vi "HFRR ADV v04.vi"() -> ()   [LabVIEW 2025] (continued)
                w1869 = FALSE ("autostrtflg")
                n931 = local write "autostrtflg"(w1869) -> ()
                n932 = local write "autostart"(w1869) -> ()
                n933 = local write "RUN"(TRUE ("RUN")) -> ()
                n934 = local write "String 14"(" Running....." ("String 14")) -> ()
              }
            }
          }
          frame Enabled {
          }
        }
        n935 = Insert Into Array(array=string[] ["Air Temperature has reached set value,", "Humidity has reached set value,", "Sample Temperaturehas reached set value,", ""], index=0, new element="") -> (w1820:string[])
        n936 = for {
          tunnel: w1821 -> [w1919] mode=indexing
          tunnel: w1820 -> [w1918]
          shift-right: [w1915] -> w1819
          shift-left: "" -> [w1917]
          n937 = Index Array(array=w1918, index=w1919) -> (element=w1916:string)
          n938 = Concatenate Strings(w1916, w1917) -> (w1915:string)
        }
        n939 = local write "autostart 2"(w1819) -> ()
      }
      frame 1 {
        # "Elapsed time\ncof\nstroke\nAir temp\nTemp\nHumidity"
        n940 = case shown="True" "OPEN 4" {
          frame False {
          }
          frame True {
            (unwired) 0  # existing file
            w2428 = "Choose a datalog file to open"  # prompt
            n941 = local write "OPEN 4"(FALSE ("OPEN 1")) -> ()
            n942 = String To Path(string="C:\\LAB-IQ-NXT\\Data\\") -> (path=w2413:path)
            n943 = File Dialog(6:"*.dgf" ("pattern"), 7:w2428, 11:w2413) -> (0:w2411:errorcluster, 3:w2419:path)  [unwired: 4 in, 2 out]
            n944 = Unbundle(w2411) -> ()  [unwired: 3 out]
            n945 = Path To String(path=w2419) -> (string=w2414:string)
            "string1 4" <- w2414
            n946 = Match Pattern(string=w2414, regular expression=".dgf" ("substring (\"\")")) -> (before substring=w2424:string)  [unwired: 1 in, 3 out]
            n947 = Concatenate Strings(w2424, ".duf" ("Substring")) -> (w2421:string)
            n948 = String To Path(string=w2421) -> (path=w2425:path)
            n949 = call <vilib>:"Read Characters From File.vi"("file path (dialog if empty)"=w2425, "start of read offset (chars.:0)"=60 ("start of read offset (chars.: 0)")) -> ("character string"=→"String Control 8":string)  [unwired: 4 in, 3 out]
            n950 = Strip Path(path=w2419) -> (name=w2417:string)  [unwired: 1 out]
            n951 = Match Pattern(string=w2417, regular expression=".dgf") -> (before substring=→"String Control 7":string)  [unwired: 1 in, 3 out]
          }
        }
        n952 = case shown="True" "OPEN 3" {
          frame False {
          }
          frame True {
            (unwired) 0  # existing file
            w2410 = "Choose a datalog file to open"  # prompt
            n953 = local write "OPEN 3"(FALSE ("OPEN 1")) -> ()
            n954 = String To Path(string="C:\\LAB-IQ-NXT\\Data\\") -> (path=w2395:path)
            n955 = File Dialog(6:"*.dgf" ("pattern"), 7:w2410, 11:w2395) -> (0:w2393:errorcluster, 3:w2401:path)  [unwired: 4 in, 2 out]
            n956 = Unbundle(w2393) -> ()  [unwired: 3 out]
            n957 = Path To String(path=w2401) -> (string=w2396:string)
            "string1 3" <- w2396
            n958 = Match Pattern(string=w2396, regular expression=".dgf" ("substring (\"\")")) -> (before substring=w2406:string)  [unwired: 1 in, 3 out]
            n959 = Concatenate Strings(w2406, ".duf" ("Substring")) -> (w2403:string)
            n960 = String To Path(string=w2403) -> (path=w2407:path)
            n961 = call <vilib>:"Read Characters From File.vi"("file path (dialog if empty)"=w2407, "start of read offset (chars.:0)"=60 ("start of read offset (chars.: 0)")) -> ("character string"=→"String Control 6":string)  [unwired: 4 in, 3 out]
            n962 = Strip Path(path=w2401) -> (name=w2399:string)  [unwired: 1 out]
            n963 = Match Pattern(string=w2399, regular expression=".dgf") -> (before substring=→"String Control 5":string)  [unwired: 1 in, 3 out]
          }
        }
        n964 = case shown="True" "OPEN 2" {
          frame False {
          }
          frame True {
            (unwired) 0  # existing file
            w2392 = "Choose a datalog file to open"  # prompt
            n965 = local write "OPEN 2"(FALSE ("OPEN 1")) -> ()
            n966 = String To Path(string="C:\\LAB-IQ-NXT\\Data\\") -> (path=w2377:path)
            n967 = File Dialog(6:"*.dgf" ("pattern"), 7:w2392, 11:w2377) -> (0:w2375:errorcluster, 3:w2383:path)  [unwired: 4 in, 2 out]
            n968 = Unbundle(w2375) -> ()  [unwired: 3 out]
            n969 = Path To String(path=w2383) -> (string=w2378:string)
            "string1 2" <- w2378
            n970 = Match Pattern(string=w2378, regular expression=".dgf" ("substring (\"\")")) -> (before substring=w2389:string)  [unwired: 1 in, 3 out]
            n971 = Concatenate Strings(w2389, ".duf" ("Substring")) -> (w2386:string)
            n972 = String To Path(string=w2386) -> (path=w2384:path)
            n973 = call <vilib>:"Read Characters From File.vi"("file path (dialog if empty)"=w2384, "start of read offset (chars.:0)"=60 ("start of read offset (chars.: 0)")) -> ("character string"=→"String Control 4":string)  [unwired: 4 in, 3 out]
            n974 = Strip Path(path=w2383) -> (name=w2381:string)  [unwired: 1 out]
            n975 = Match Pattern(string=w2381, regular expression=".dgf") -> (before substring=→"String Control 3":string)  [unwired: 1 in, 3 out]
          }
        }
        n976 = case shown="True" "OPEN 1" {
          frame False {
          }
          frame True {
            (unwired) 0  # existing file
            w2374 = "Choose a datalog file to open"  # prompt
            n977 = local write "OPEN 1"(FALSE ("OPEN 1")) -> ()
            n978 = String To Path(string="C:\\LAB-IQ-NXT\\Data\\") -> (path=w2359:path)
            n979 = File Dialog(6:"*.dgf" ("pattern"), 7:w2374, 11:w2359) -> (0:w2357:errorcluster, 3:w2365:path)  [unwired: 4 in, 2 out]
            n980 = Unbundle(w2357) -> ()  [unwired: 3 out]
            n981 = Path To String(path=w2365) -> (string=w2360:string)
            "string1" <- w2360
            n982 = Match Pattern(string=w2360, regular expression=".dgf" ("substring (\"\")")) -> (before substring=w2370:string)  [unwired: 1 in, 3 out]
            n983 = Concatenate Strings(w2370, ".duf" ("Substring")) -> (w2366:string)
            n984 = String To Path(string=w2366) -> (path=w2371:path)
            n985 = call <vilib>:"Read Characters From File.vi"("file path (dialog if empty)"=w2371, "start of read offset (chars.:0)"=60 ("start of read offset (chars.: 0)")) -> ("character string"=→"String Control 2":string)  [unwired: 4 in, 3 out]
            n986 = Strip Path(path=w2365) -> (name=w2364:string)  [unwired: 1 out]
            n987 = Match Pattern(string=w2364, regular expression=".dgf") -> (before substring=→"String Control":string)  [unwired: 1 in, 3 out]
          }
        }
        n988 = case shown="True" "RSTV1 4" {
          frame False {
          }
          frame True {
            n989 = property on="Stroke" class="XYGraph (strict)"("Y Scale.Display Format:Precision"=u8 2 ("Y Scale.Format & Precision:Precision")) -> ()  [unwired: 2 in, 2 out]
            n990 = property on="Stroke" class="XYGraph (strict)"("X Scale.Range:Minimum"=0.0 ("Y Scale.Range:Maximum"), "X Scale.Range:Maximum"=75.0 ("X Scale.Range:Minimum"), "Y Scale.Range:Minimum"=0.98, "Y Scale.Range:Maximum"=1.02) -> ()  [unwired: 2 in, 2 out]
          }
        }
        n991 = case shown="True" "rstv2" {
          frame False {
          }
          frame True {
            n992 = property on="Coefficient Of Friction" class="XYGraph (strict)"("X Scale.Range:Minimum"=0.0 ("Y Scale.Range:Maximum"), "X Scale.Range:Maximum"=75.0, "Y Scale.Range:Minimum"=0.0, "Y Scale.Range:Maximum"=1.0 ("X Scale.Range:Minimum")) -> ()  [unwired: 2 in, 2 out]
            n993 = property on="Coefficient Of Friction" class="XYGraph (strict)"("Y Scale.Display Format:Precision"=u8 3 ("Y Scale.Format & Precision:Precision")) -> ()  [unwired: 2 in, 2 out]
          }
        }
        n994 = case shown="True" "RSTV1 3" {
          frame False {
          }
          frame True {
            n995 = property on="Air Temperature" class="XYGraph (strict)"("X Scale.Range:Minimum"=0.0 ("Y Scale.Range:Minimum"), "X Scale.Range:Maximum"=75.0 ("Y Scale.Range:Maximum"), "Y Scale.Range:Minimum"=20.0 ("X Scale.Range:Minimum"), "Y Scale.Range:Maximum"=26.0 ("X Scale.Range:Maximum")) -> ()  [unwired: 2 in, 2 out]
            n996 = property on="Air Temperature" class="XYGraph (strict)"("Y Scale.Display Format:Precision"=u8 2 ("Y Scale.Format & Precision:Precision")) -> ()  [unwired: 2 in, 2 out]
          }
        }
        n997 = case shown="True" "RST CP" {
          frame False {
          }
          frame True {
            n998 = property on="Sample Temperature" class="XYGraph (strict)"("X Scale.Range:Minimum"=0.0, "X Scale.Range:Maximum"=75.0, "Y Scale.Range:Minimum"=58.0, "Y Scale.Range:Maximum"=62.0) -> ()  [unwired: 2 in, 2 out]
            n999 = property on="Sample Temperature" class="XYGraph (strict)"("Y Scale.Display Format:Precision"=u8 2 ("Y Scale.Format & Precision:Precision")) -> ()  [unwired: 2 in, 2 out]
          }
        }
        n1000 = case shown="True" "RST CP 2" {
          frame False {
          }
          frame True {
            n1001 = property on="XY Graph 13" class="XYGraph (strict)"("X Scale.Range:Minimum"=0.0, "X Scale.Range:Maximum"=75.0, "Y Scale.Range:Minimum"=0.0, "Y Scale.Range:Maximum"=100.0) -> ()  [unwired: 2 in, 2 out]
            n1002 = property on="XY Graph 13" class="XYGraph (strict)"("Y Scale.Display Format:Precision"=u8 0 ("Y Scale.Format & Precision:Precision")) -> ()  [unwired: 2 in, 2 out]
          }
        }
        n1003 = case shown="True" "RSTV1 2" {
          frame False {
          }
          frame True {
            n1004 = property on="Humidity" class="XYGraph (strict)"("X Scale.Range:Minimum"=0.0, "X Scale.Range:Maximum"=75.0, "Y Scale.Range:Minimum"=48.0, "Y Scale.Range:Maximum"=58.0) -> ()  [unwired: 2 in, 2 out]
            n1005 = property on="Humidity" class="XYGraph (strict)"("Y Scale.Display Format:Precision"=u8 0 ("Y Scale.Format & Precision:Precision")) -> ()  [unwired: 2 in, 2 out]
          }
        }
        n1006 = case shown="True" "RST CP 3" {
          frame False {
          }
          frame True {
            n1007 = property on="Air Temp vs Rh" class="XYGraph (strict)"("X Scale.Range:Minimum"=18.0, "X Scale.Range:Maximum"=28.0 ("X Scale.Range:Minimum"), "Y Scale.Range:Minimum"=30.0 ("X Scale.Range:Minimum"), "Y Scale.Range:Maximum"=70.0 ("X Scale.Range:Minimum")) -> ()  [unwired: 2 in, 2 out]
          }
        }
      }
      frame 2 {
        # "Elapsed time\ncof\nstroke\nmean pos\nTemp\nHumidity"
        n1008 = case shown="True" "Export" {
          frame False {
          }
          frame True {
            w2558 = "                                      " ("string")
            w2560 = "\r"
            (unwired) i16 6 ("width (-)")
            w2637 = "\r"
            w2569 = "\r"
            n1009 = local read "Sample ID"() -> (w2644:string)
            n1010 = local read "Temperature after test 2"() -> (w2631:dbl)
            n1011 = local read "Test Date"() -> (w2643:string)
            n1012 = local read "String 45"() -> (w2557:string)
            n1013 = local read "String 32"() -> (w2641:string)
            n1014 = local read "String 31"() -> (w2642:string)
            n1015 = local read "String 38"() -> (w2579:string)
            n1016 = local read "Humidity after test 2"() -> (w2627:dbl)
            n1017 = local read "s.NO"() -> (w2559:string)
            n1018 = local read "String 36"() -> (w2582:string)
            n1019 = local read "Temperature before test 2"() -> (w2626:dbl)
            n1020 = local read "String 37"() -> (w2585:string)
            n1021 = local read "AVP 2"() -> (w2624:dbl)
            n1022 = local read "HCF 2"() -> (w2635:dbl)
            n1023 = local read "MWSD 2"() -> (w2623:dbl)
            n1024 = local read "String 35"() -> (w2589:string)
            n1025 = local write "Export"(FALSE ("Export")) -> ()
            n1026 = local read "Humidity before test 2"() -> (w2612:dbl)
            n1027 = Concatenate Strings("7," ("string"), w2579) -> (w2580:string)
            n1028 = Concatenate Strings("6," ("string"), w2582) -> (w2583:string)
            n1029 = local read "S 39"() -> (w2590:string)
            n1030 = Concatenate Strings("5," ("string"), w2585) -> (w2586:string)
            n1031 = local read "String 34"() -> (w2594:string)
            n1032 = Concatenate Strings("4," ("string"), w2589) -> (w2588:string)
            n1033 = Concatenate Strings("3," ("string"), w2590) -> (w2592:string)
            n1034 = local read "S 38"() -> (w2597:string)
            n1035 = Number To Fractional String(number=w2635, width (-)=i16 6, precision (6)=i16 2) -> (F-format string=w2636:string)  [unwired: 1 in]
            n1036 = Number To Fractional String(number=w2623, width (-)=i16 6, precision (6)=i16 2) -> (F-format string=w2621:string)  [unwired: 1 in]
            n1037 = Number To Fractional String(number=w2624, width (-)=i16 6, precision (6)=i16 2) -> (F-format string=w2622:string)  [unwired: 1 in]
            n1038 = Number To Fractional String(number=w2631, width (-)=i16 6, precision (6)=i16 2) -> (F-format string=w2630:string)  [unwired: 1 in]
            n1039 = Number To Fractional String(number=w2627, width (-)=i16 6, precision (6)=i16 2) -> (F-format string=w2625:string)  [unwired: 1 in]
            n1040 = Number To Fractional String(number=w2626, width (-)=i16 6, precision (6)=i16 2) -> (F-format string=w2632:string)  [unwired: 1 in]
            n1041 = Number To Fractional String(number=w2612, width (-)=i16 6, precision (6)=i16 2) -> (F-format string=w2611:string)  [unwired: 1 in]
            n1042 = local read "String 39"() -> (w2576:string)
            n1043 = Concatenate Strings("2," ("string"), w2594) -> (w2593:string)
            n1044 = local read "WS1.4 2"() -> (w2639:dbl)
            n1045 = Concatenate Strings(w2569, "," ("string"), w2557, w2559, w2558, w2641, w2644, w2558, w2642, w2643, w2569) -> (w2567:string)
            n1046 = Concatenate Strings("1," ("string"), w2597) -> (w2596:string)
            n1047 = Concatenate Strings("8," ("string"), w2576) -> (w2577:string)
            n1048 = Number To Fractional String(number=w2639, precision (6)=i16 2) -> (F-format string=w2640:string)  [unwired: 2 in]
            n1049 = Concatenate Strings(w2637, w2596, w2611, w2637, w2593, w2632, w2637, w2592, w2625, w2637, w2588, w2630, w2637, w2586, w2621, w2637, w2583, w2622, w2637, w2580, w2636, w2637, w2577, w2640) -> (w2599:string)
            n1050 = Concatenate Strings("S.No," ("string"), "                                       Parameters" ("string")) -> (w2570:string)
            n1051 = local read "TITTLE"() -> (w2565:string)
            n1052 = local read "String 33"() -> (w2574:string)
            n1053 = local read "Tested by"() -> (w2573:string)
            n1054 = Concatenate Strings("=" ("string"), w2565) -> (w2564:string)
            n1055 = local read "String 29"() -> (w2606:string)
            n1056 = Concatenate Strings("," ("string"), "                                                                             " ("string")) -> (w2562:string)
            n1057 = Concatenate Strings(w2564, w2560, w2567, w2560, w2570, w2599, w2560, w2562, w2574, w2573) -> (→"export":string)
            n1058 = Match Pattern(string=w2606, regular expression=".dwm") -> (before substring=w2602:string)  [unwired: 1 in, 3 out]
            "before substring" <- w2602
            n1059 = case shown="\"xlx\"" "Select File Type" {
              tunnel: w2602 -> [w2647 w2649 w2651]
              tunnel: [w2645 w2650 w2652] -> w2601
              frame "xlx" {
                n1060 = Concatenate Strings(w2647, ".xls" ("string")) -> (w2645:string)
              }
              frame "csv" {
                n1061 = Concatenate Strings(w2649, ".csv" ("string")) -> (w2650:string)
              }
              frame "txt" {
                n1062 = Concatenate Strings(w2651, ".txt" ("string")) -> (w2652:string)
              }
            }
            n1063 = String To Path(string=w2601) -> (path=w2608:path)
            n1064 = local read "export"() -> (w2603:string)
            n1065 = call <vilib>:"Write Characters To File.vi"("append to file? (new file:F)"=FALSE, "character string"=w2603, "file path (dialog if empty)"=w2608) -> ()  [unwired: 2 in, 1 out]
          }
        }
        n1066 = case shown="True" "OK Button 16" {
          frame False {
          }
          frame True {
            n1067 = stacked-sequence {
              frame #0 {
                n1068 = local read "Numeric 16"() -> (w2767:i32)
                n1069 = local write "Numeric 10"(w2767) -> ()
              }
              frame #1 {
                n1070 = local read "String 29"() -> (w2771:string)
                n1071 = String To Path(string=w2771) -> (path=w2770:path)
                n1072 = local read "S.NO"() -> (→"s.NO":string)
                n1073 = Open/Create/Replace File "Open File"(file path (use dialog)=w2770) -> (refnum out=w2772:refnum<file>)  [unwired: 5 in, 2 out]
                n1074 = for {
                  N: 16 -> [_]
                  tunnel: w2772 -> [w2779]
                  i -> [w2775]
                  (unwired) TRUE ("line mode (F)")
                  n1075 = Read from Text File "Read File"(file (use dialog)=w2779) -> (text=w2773:string)  [unwired: 3 in, 3 out]
                  n1076 = Match Pattern(string=w2773, regular expression="(") -> (after substring=w2778:string)  [unwired: 1 in, 3 out]
                  n1077 = Match Pattern(string=w2778, regular expression=")") -> (before substring=w2774:string)  [unwired: 1 in, 3 out]
                  n1078 = case shown="1" w2775 {
                    tunnel: w2774 -> [w2780 w2781 _ _ w2782 w2783 w2784 w2786 w2788 w2790 w2792 w2794 w2796 w2798 _]
                    tunnel: w2773 -> [_ _ _ _ _ _ _ _ _ _ _ _ _ _ _]
                    frame 0 {
                      "TITTLE" <- w2780
                    }
                    frame 1 {
                      "Sample ID" <- w2781
                    }
                    frame 2 {
                    }
                    frame 3 {
                    }
                    frame 4 {
                      "Test Date" <- w2782
                    }
                    frame 5 {
                      "Tested by" <- w2783
                    }
                    frame 6 {
                      n1079 = Fract/Exp String To Number(string=w2784) -> (number=→"Humidity before test 2":dbl)  [unwired: 3 in, 1 out]
                    }
                    frame 7 {
                      n1080 = Fract/Exp String To Number(string=w2786) -> (number=→"Temperature before test 2":dbl)  [unwired: 3 in, 1 out]
                    }
                    frame 8 {
                      n1081 = Fract/Exp String To Number(string=w2788) -> (number=→"Humidity after test 2":dbl)  [unwired: 3 in, 1 out]
                    }
                    frame 9 {
                      n1082 = Fract/Exp String To Number(string=w2790) -> (number=→"Temperature after test 2":dbl)  [unwired: 3 in, 1 out]
                    }
                    frame 10 {
                      n1083 = Fract/Exp String To Number(string=w2792) -> (number=→"MWSD 2":dbl)  [unwired: 3 in, 1 out]
                    }
                    frame 11 {
                      n1084 = Fract/Exp String To Number(string=w2794) -> (number=→"AVP 2":dbl)  [unwired: 3 in, 1 out]
                    }
                    frame 12 {
                      n1085 = Fract/Exp String To Number(string=w2796) -> (number=→"HCF 2":dbl)  [unwired: 3 in, 1 out]
                    }
                    frame 13 {
                      n1086 = Fract/Exp String To Number(string=w2798) -> (number=→"WS1.4 2":dbl)  [unwired: 3 in, 1 out]
                    }
                    frame 14, Default {
                    }
                  }
                }
              }
              frame #2 {
              }
            }
            n1087 = local write "OK Button 16"(FALSE ("OK Button 13")) -> ()
          }
        }
        n1088 = call <vilib>:"Query Available Printers.vi"() -> ("system configured printers"=w2443:string[])  [unwired: 9 in, 2 out]
        "System Configured Printers 2" <- w2443
        n1089 = Index Array(array=w2443, index="Select Printer 3") -> (element=w2445:string)
        "Selected Printer" <- w2445
        n1090 = local read "OK Button 16"() -> (w2439:bool)
        n1091 = case shown="True" "Print" {
          tunnel: w2445 -> [_ w2736]
          frame False {
          }
          frame True {
            (unwired) i16 6 ("width (-)")
            (unwired) "TESTED BY : "
            (unwired) "TESTED DATE :"
            (unwired) "SAMPLE ID : "
            (unwired) "SAMPLE DESIGN : "
            w2694 = "\r"
            w2711 = "\r"
            # "add image"
            n1092 = local read "String 45"() -> (w2654:string)
            n1093 = local read "Sample ID"() -> (w2684:string)
            n1094 = local read "Tested by"() -> (w2687:string)
            n1095 = local read "Test Date"() -> (w2685:string)
            n1096 = local read "String 32"() -> (w2689:string)
            n1097 = local read "String 31"() -> (w2688:string)
            n1098 = local read "String 33"() -> (w2690:string)
            n1099 = local read "s.NO"() -> (w2655:string)
            n1100 = call <vilib>:"New Report.vi"("report type"=enum16{"Standard Report", "HTML"}."Standard Report") -> ("report out"=w2734:refnum<class "NI_report.lvclass">, "error out"=w2733:errorcluster)  [unwired: 13 in]
            n1101 = local read "TITTLE"() -> (w2686:string)
            n1102 = call-dynamic "Set Report Header Text.vi"("report in"=w2734, "center header text"=w2686, "error in (no error)"=w2733) -> ("report out"=w2705:refnum<class "NI_report.lvclass">, "error out"=w2706:errorcluster)  [unwired: 11 in]
            n1103 = Concatenate Strings(w2711, w2654, w2655, w2711, w2689, w2684, w2711, w2688, w2685, w2711, w2690, w2687, w2711) -> (w2704:string)
            "test by" <- w2704
            n1104 = local read "Temperature after test 2"() -> (w2700:dbl)
            n1105 = local read "String 38"() -> (w2660:string)
            n1106 = local read "Humidity after test 2"() -> (w2709:dbl)
            n1107 = local read "String 36"() -> (w2664:string)
            n1108 = local read "Temperature before test 2"() -> (w2710:dbl)
            n1109 = local read "String 37"() -> (w2667:string)
            n1110 = local read "AVP 2"() -> (w2713:dbl)
            n1111 = local read "HCF 2"() -> (w2696:dbl)
            n1112 = local read "MWSD 2"() -> (w2714:dbl)
            n1113 = local read "String 35"() -> (w2669:string)
            n1114 = call-poly <vilib>:"Append Report Text.vi"("report in"=w2705, "text"=w2704, "error in (no error)"=w2706) -> ("report out"=w2708:refnum<class "NI_report.lvclass">, "error out"=w2707:errorcluster)  [unwired: 9 in, 2 out]
            n1115 = local read "Humidity before test 2"() -> (w2725:dbl)
            n1116 = Concatenate Strings("7)" ("string"), w2660) -> (w2661:string)
            n1117 = local read "S 39"() -> (w2672:string)
            n1118 = local read "String 34"() -> (w2674:string)
            n1119 = Concatenate Strings("6)" ("string"), w2664) -> (w2663:string)
            n1120 = Concatenate Strings("5)" ("string"), w2667) -> (w2666:string)
            n1121 = Concatenate Strings("4)" ("string"), w2669) -> (w2670:string)
            n1122 = Concatenate Strings("3)" ("string"), w2672) -> (w2673:string)
            n1123 = local read "S 38"() -> (w2679:string)
            n1124 = Concatenate Strings("2)" ("string"), w2674) -> (w2675:string)
            n1125 = Number To Fractional String(number=w2696, width (-)=i16 6, precision (6)=i16 2) -> (F-format string=w2695:string)  [unwired: 1 in]
            n1126 = Number To Fractional String(number=w2714, width (-)=i16 6, precision (6)=i16 2) -> (F-format string=w2716:string)  [unwired: 1 in]
            n1127 = Number To Fractional String(number=w2713, width (-)=i16 6, precision (6)=i16 2) -> (F-format string=w2715:string)  [unwired: 1 in]
            n1128 = Number To Fractional String(number=w2700, width (-)=i16 6, precision (6)=i16 2) -> (F-format string=w2701:string)  [unwired: 1 in]
            n1129 = Number To Fractional String(number=w2709, width (-)=i16 6, precision (6)=i16 2) -> (F-format string=w2712:string)  [unwired: 1 in]
            n1130 = Number To Fractional String(number=w2710, width (-)=i16 6, precision (6)=i16 2) -> (F-format string=w2699:string)  [unwired: 1 in]
            n1131 = Number To Fractional String(number=w2725, width (-)=i16 6, precision (6)=i16 2) -> (F-format string=w2730:string)  [unwired: 1 in]
            n1132 = call-poly <vilib>:"Append Report Text.vi"("report in"=w2708, "error in (no error)"=w2707) -> ("report out"=w2729:refnum<class "NI_report.lvclass">, "error out"=w2727:errorcluster)  [unwired: 10 in, 2 out]
            n1133 = local read "String 39"() -> (w2657:string)
            n1134 = local read "WS1.4 2"() -> (w2692:dbl)
            n1135 = Concatenate Strings("1)" ("string"), w2679) -> (w2678:string)
            n1136 = Concatenate Strings("8)" ("string"), w2657) -> (w2658:string)
            n1137 = Number To Fractional String(number=w2692, precision (6)=i16 2) -> (F-format string=w2691:string)  [unwired: 2 in]
            n1138 = Concatenate Strings(w2694, w2678, w2730, w2694, w2675, w2699, w2694, w2673, w2712, w2694, w2670, w2701, w2694, w2666, w2716, w2694, w2663, w2715, w2694, w2661, w2695, w2694, w2658, w2691) -> (w2682:string)
            "export 2" <- w2682
            n1139 = call-poly <vilib>:"Append Report Text.vi"("report in"=w2729, "text"=w2682, "error in (no error)"=w2727) -> ("report out"=w2728:refnum<class "NI_report.lvclass">, "error out"=w2726:errorcluster)  [unwired: 9 in, 2 out]
            n1140 = call-dynamic "Print Report.vi"("report in"=w2728, "printer name (default)"=w2736, "error in (no error)"=w2726) -> ("report out"=w2738:refnum<class "NI_report.lvclass">, "error out"=w2739:errorcluster)  [unwired: 11 in]
            n1141 = local read "test by"() -> (w2681:string)
            n1142 = local read "TITTLE"() -> (w2683:string)
            n1143 = local write "Print"(FALSE ("Print FF")) -> ()
            n1144 = call-dynamic "Dispose Report.vi"("report in"=w2738, "error in (no error)"=w2739) -> ()  [unwired: 13 in, 1 out]
            n1145 = Concatenate Strings(w2683, w2682, w2681) -> (→"output":string)
          }
        }
        n1146 = case shown="True" w2439 {
          frame False {
          }
          frame True {
            n1147 = flat-sequence {
              frame #0 {
              }
              frame #1 {
                n1148 = Wait (ms)(milliseconds to wait=u32 100) -> ()  [unwired: 1 out]
              }
              frame #2 {
                n1149 = local write "OK Button 16"(FALSE ("Print 3")) -> ()
              }
            }
          }
        }
        n1150 = case shown="True" "OK Button 17" {
          frame False {
          }
          frame True {
            (unwired) 0  # existing file
            w2753 = "Choose a datalog file to open"  # prompt
            n1151 = local read "String"() -> (w2748:string)
            n1152 = local write "OK Button 17"(FALSE ("OK Button 17")) -> ()
            n1153 = String To Path(string=w2748) -> (path=w2749:path)
            n1154 = File Dialog(6:"*.duf" ("pattern"), 7:w2753, 11:w2749) -> (0:w2740:errorcluster, 3:w2759:path)  [unwired: 4 in, 2 out]
            n1155 = Unbundle(w2740) -> ()  [unwired: 3 out]
            n1156 = Open/Create/Replace File "Open File"(file path (use dialog)=w2759) -> (refnum out=w2751:refnum<file>)  [unwired: 5 in, 2 out]
            n1157 = Path To String(path=w2759) -> (string=w2742:string)
            n1158 = while {
              tunnel: w2751 -> [w2763]
              i -> [w2760]
              stop <- w2761 continue-if-true
              (unwired) TRUE ("line mode (F)")
              n1159 = local write "Numeric 16"(w2760) -> ()
              n1160 = Read from Text File "Read File"(file (use dialog)=w2763) -> (text=w2762:string)  [unwired: 3 in, 3 out]
              n1161 = String Length(string=w2762) -> (length=w2765:i32)
              n1162 = Greater?(x=w2765, y=1) -> (0:w2761:bool)
            }
            n1163 = local write "String 29"(w2742) -> ()
            n1164 = Match Pattern(string=w2742, regular expression=".dwm" ("substring (\"\")")) -> (before substring=w2743:string)  [unwired: 1 in, 3 out]
            "String Indicator 3" <- w2743
            n1165 = Search and Replace String(input string=w2742, search string=".duf", replace string=".dgf" ("replace string (\"\")")) -> (result string=→"String Indicator 4":string)  [unwired: 5 in, 3 out]
            n1166 = String To Path(string=w2743) -> (path=w2750:path)
            "path" <- w2750
            n1167 = Strip Path(path=w2759) -> (name=w2757:string)  [unwired: 1 out]
            n1168 = call <vilib>:"Read Characters From File.vi"("file path (dialog if empty)"=w2750, "start of read offset (chars.:0)"=60 ("start of read offset (chars.: 0)")) -> ("character string"=→"String Indicator 2":string)  [unwired: 4 in, 3 out]
            n1169 = Match Pattern(string=w2757, regular expression=".dwm") -> (before substring=w2741:string)  [unwired: 1 in, 3 out]
            "String Indicator" <- w2741
            n1170 = local write "TITTLE 2"(w2741) -> ()
          }
        }
        n1171 = case shown="True" "Print 2" {
          frame False {
          }
          frame True {
            n1172 = flat-sequence {
              frame #0 {
                n1173 = local read "s.NO"() -> (→"s.NO 2":string)
                n1174 = local read "Sample ID  3"() -> (→"Sample ID  6":string)
                n1175 = local read "Sample ID  4"() -> (→"Sample ID  7":string)
                n1176 = local read "Sample ID"() -> (→"Sample ID  2":string)
                n1177 = local read "Tested by"() -> (→"Tested by 2":string)
                n1178 = local read "Test Date"() -> (→"Test Date 2":string)
                n1179 = Wait (ms)(milliseconds to wait=u32 20) -> ()  [unwired: 1 out]
                n1180 = local read "Humidity after test 3"() -> (→"Humidity after test 4":dbl)
                n1181 = local read "Ref A Test Date :"() -> (→"TITTLE 4":string)
                n1182 = local read "Temperature before test 3"() -> (w2463:dbl)
                n1183 = local read "Temperature before test 3"() -> (→"Temperature after test 5":dbl)
                n1184 = local read "Temperature after test 3"() -> (→"Temperature after test 4":dbl)
                n1185 = local read "Humidity before test 3"() -> (→"Humidity before test 4":dbl)
                n1186 = local write "Temperature before test 3"(w2463) -> ()
                n1187 = local read "image data"() -> (w2454:T11)
                n1188 = String To Path(string="C:\\LAB-IQ-NXT\\im\\Temp_resized.jpg") -> (path=w2455:path)
                "path 2" <- w2455
                n1189 = call <vilib>:"Write JPEG File.vi"("image data"=w2454, "path to JPEG file"=w2455) -> ()  [unwired: 8 in, 2 out]
                "Ref A Test Date :" <- "Ref A Test Date :"
                "Ref B Test Date :" <- "Ref B Test Date :"
                "Ref B Scar Value :" <- "Ref B Scar Value :"
                "Ref A Scar Value :" <- "Ref A Scar Value :"
              }
              frame #1 {
                (unwired) HTML_Report_Image_Alignment."MIDDLE" ("alignment (default)")
                w2491 = u16 0 items=["portrait", "landscape"] ("orientation (portrait)")
                (unwired) HTML_Report_Image_Alignment."ABSMIDDLE" ("alignment (default)")
                (unwired) "TESTED BY : "
                (unwired) "TESTED DATE :"
                (unwired) "SAMPLE ID : "
                (unwired) "SAMPLE DESIGN : "
                w2524 = "\r"
                # "add image"
                n1190 = local read "Sample ID  2"() -> (w2517:string)
                n1191 = local read "Wear Scar X"() -> (w2489:dbl)
                "Length ( microns ) 2" <- w2489
                n1192 = local read "Wear Scar Y"() -> (w2488:dbl)
                "Wear Scar Y ( microns ) :" <- w2488
                n1193 = local read "Tested by 2"() -> (w2519:string)
                n1194 = local read "Test Date 2"() -> (w2518:string)
                n1195 = local read "String 46"() -> (w2515:string)
                n1196 = local read "String 48"() -> (w2521:string)
                n1197 = local read "String 47"() -> (w2520:string)
                n1198 = local read "String 49"() -> (w2522:string)
                n1199 = Wait (ms)(milliseconds to wait=u32 20) -> ()  [unwired: 1 out]
                n1200 = local read "String 10"() -> (w2475:string)
                n1201 = local read "s.NO 2"() -> (w2516:string)
                n1202 = Add(x=w2489, y=w2488) -> (x+y=w2487:dbl)
                n1203 = call <vilib>:"New Report.vi"("report type"=enum16{"Standard Report", "HTML"}."HTML") -> ("report out"=w2495:refnum<class "NI_report.lvclass">, "error out"=w2493:errorcluster)  [unwired: 13 in]
                n1204 = Concatenate Strings(w2524, w2515, w2516, w2524, w2521, w2517, w2524, w2520, w2518, w2524, w2522, w2519, w2524) -> (→"test by 2":string)
                n1205 = Divide(x=w2487, y=2.0) -> (x/y=→"Mean Wear ( microns) :":dbl)
                n1206 = Concatenate Strings("C:\\LAB-IQ-NXT\\Data\\" ("string"), w2475, ".jpg" ("string")) -> ()  [unwired: 1 out]
                n1207 = call-dynamic "Set Report Orientation.vi"("report in"=w2495, "orientation (portrait)"=w2491, "error in (no error)"=w2493) -> ("report out"=w2494:refnum<class "NI_report.lvclass">, "error out"=w2492:errorcluster)  [unwired: 11 in]
                n1208 = for {
                  N: 5 -> [_]
                  tunnel: w2494 -> [w2545]
                  tunnel: [w2544] -> w2473
                  tunnel: w2492 -> [w2543]
                  tunnel: [w2542] -> w2472
                  n1209 = call-dynamic "Set Report Tab Width.vi"("report in"=w2545, "error in (no error)"=w2543) -> ("report out"=w2544:refnum<class "NI_report.lvclass">, "error out"=w2542:errorcluster)  [unwired: 12 in]
                }
                n1210 = local read "TITTLE"() -> (w2490:string)
                n1211 = call-dynamic "Set Report Header Text.vi"("report in"=w2473, "center header text"=w2490, "error in (no error)"=w2472) -> ("report out"=w2511:refnum<class "NI_report.lvclass">, "error out"=w2510:errorcluster)  [unwired: 11 in]
                n1212 = for {
                  N: 1 -> [_]
                  tunnel: [w2549] -> w2497
                  tunnel: [w2548] -> w2496
                  tunnel: w2511 -> [w2547]
                  tunnel: w2510 -> [w2546]
                  n1213 = call-dynamic "New Report Line.vi"("report in"=w2547, "error in (no error)"=w2546) -> ("report out"=w2549:refnum<class "NI_report.lvclass">, "error out"=w2548:errorcluster)  [unwired: 12 in]
                }
                n1214 = for {
                  N: 2 -> [_]
                  tunnel: [w2541] -> w2503
                  tunnel: [w2540] -> w2502
                  tunnel: w2497 -> [w2539]
                  tunnel: w2496 -> [w2538]
                  n1215 = call-dynamic "New Report Line.vi"("report in"=w2539, "error in (no error)"=w2538) -> ("report out"=w2541:refnum<class "NI_report.lvclass">, "error out"=w2540:errorcluster)  [unwired: 12 in]
                }
                n1216 = for {
                  N: 25 -> [_]
                  tunnel: w2503 -> [w2537]
                  tunnel: w2502 -> [w2535]
                  tunnel: [w2536] -> w2506
                  tunnel: [w2534] -> w2505
                  n1217 = call-dynamic "Set Report Tab Width.vi"("report in"=w2537, "error in (no error)"=w2535) -> ("report out"=w2536:refnum<class "NI_report.lvclass">, "error out"=w2534:errorcluster)  [unwired: 12 in]
                }
                n1218 = control-ref of="Tab Control 9"() -> (w2501:refnum<vi>)
                n1219 = call-dynamic "Append Control Image to Report.vi"("report in"=w2506, "alignment (default)"=HTML_Report_Image_Alignment."ABSMIDDLE", "ctrl reference"=w2501, "error in (no error)"=w2505) -> ("report out"=w2500:refnum<class "NI_report.lvclass">, "error out"=w2499:errorcluster)  [unwired: 8 in, 2 out]
                n1220 = for {
                  N: 3 -> [_]
                  tunnel: [w2533] -> w2484
                  tunnel: [w2532] -> w2483
                  tunnel: w2500 -> [w2531]
                  tunnel: w2499 -> [w2530]
                  n1221 = call-dynamic "New Report Line.vi"("report in"=w2531, "error in (no error)"=w2530) -> ("report out"=w2533:refnum<class "NI_report.lvclass">, "error out"=w2532:errorcluster)  [unwired: 12 in]
                }
                n1222 = for {
                  N: 100 -> [_]
                  tunnel: w2484 -> [w2529]
                  tunnel: w2483 -> [w2527]
                  tunnel: [w2528] -> w2480
                  tunnel: [w2526] -> w2478
                  n1223 = call-dynamic "Set Report Tab Width.vi"("report in"=w2529, "error in (no error)"=w2527) -> ("report out"=w2528:refnum<class "NI_report.lvclass">, "error out"=w2526:errorcluster)  [unwired: 12 in]
                }
                n1224 = String To Path(string="C:\\LAB-IQ-NXT\\im\\Temp_resized.jpg") -> (path=w2470:path)
                n1225 = call-poly <vilib>:"Append Image to Report.vi"("report in"=w2480, "path or URL of image"=w2470, "error in (no error)"=w2478) -> ("report out"=w2479:refnum<class "NI_report.lvclass">, "error out"=w2477:errorcluster)  [unwired: 9 in, 2 out]
                n1226 = call-poly <vilib>:"Open HTML Report in Browser.vi"("report in"=w2479, "error in (no error)"=w2477) -> ("report out"=w2514:refnum<class "NI_report.lvclass">, "error out"=w2513:errorcluster)  [unwired: 11 in, 1 out]
                n1227 = call-dynamic "Dispose Report.vi"("report in"=w2514, "error in (no error)"=w2513) -> ()  [unwired: 13 in, 1 out]
              }
              frame #2 {
              }
              frame #3 {
                n1228 = disable-structure shown="Disabled" {
                  frame Disabled {
                    n1229 = local read "String 10"() -> (w2554:string)
                    n1230 = Concatenate Strings("C:\\LAB-IQ-NXT\\Data\\" ("string"), w2554, ".jpg" ("string")) -> (w2552:string)
                    n1231 = String To Path(string=w2552) -> (path=w2551:path)
                    n1232 = Delete(path (use dialog)=w2551) -> ()  [unwired: 4 in, 3 out]
                  }
                  frame Enabled {
                  }
                }
                n1233 = local write "Print 2"(FALSE ("Print")) -> ()
              }
            }
          }
        }
      }
    }
    n1234 = local read "OK Button 16"() -> (w816:bool)
    n1235 = Or(x=w816, y="OPEN") -> (x .or. y?=w817:bool)
    n1236 = case shown="True" w817 {
      tunnel: w816 -> [_ w852]
      frame False {
      }
      frame True {
        n1237 = stacked-sequence {
          tunnel: w852 -> [_ w919 _ _]
          frame #0 {
            w868 = "  " ("String 6")
            n1238 = local write "OPEN"(FALSE ("open")) -> ()
            n1239 = property on="OPEN" class="Bool (strict)"("Visible"=FALSE) -> ()  [unwired: 2 in, 2 out]
            n1240 = local write "String 12"(w868) -> ()
            n1241 = local write "String 6"(w868) -> ()
            n1242 = local write "String 7"(w868) -> ()
            n1243 = local write "String 8"(w868) -> ()
            n1244 = local read "OK Button 16"() -> (w853:bool)
            n1245 = case shown="True" w853 {
              tunnel: [w869 w870] -> w857
              frame False {
                n1246 = local read "string1"() -> (w869:string)
              }
              frame True {
                n1247 = local read "String Indicator 4"() -> (w870:string)
              }
            }
            n1248 = local read "string1 2"() -> (w856:string)
            n1249 = local read "string1 4"() -> (w854:string)
            n1250 = local read "string1 3"() -> (w855:string)
            n1251 = String To Path(string=w857) -> (path=w865:path)
            n1252 = String To Path(string=w856) -> (path=w864:path)
            n1253 = String To Path(string=w855) -> (path=w863:path)
            n1254 = String To Path(string=w854) -> (path=w862:path)
            n1255 = Open/Create/Replace File "Open File"(file path (use dialog)=w865) -> (refnum out=w861:refnum<file>)  [unwired: 5 in, 2 out]
            n1256 = Open/Create/Replace File "Open File"(file path (use dialog)=w864) -> (refnum out=w860:refnum<file>)  [unwired: 5 in, 2 out]
            n1257 = Open/Create/Replace File "Open File"(file path (use dialog)=w863) -> (refnum out=w859:refnum<file>)  [unwired: 5 in, 2 out]
            n1258 = Open/Create/Replace File "Open File"(file path (use dialog)=w862) -> (refnum out=w858:refnum<file>)  [unwired: 5 in, 2 out]
            n1259 = while {
              tunnel: w861 -> [w876]
              i -> [w872]
              stop <- w871 continue-if-true
              (unwired) TRUE ("line mode (F)")
              n1260 = Read from Text File "Read File"(file (use dialog)=w876) -> (text=w873:string)  [unwired: 3 in, 3 out]
              n1261 = local write "Numeric 8"(w872) -> ()
              n1262 = String Length(string=w873) -> (length=w875:i32)
              n1263 = Greater?(x=w875, y=1) -> (0:w871:bool)
            }
            n1264 = while {
              tunnel: w860 -> [w882]
              i -> [w878]
              stop <- w877 continue-if-true
              (unwired) TRUE ("line mode (F)")
              n1265 = Read from Text File "Read File"(file (use dialog)=w882) -> (text=w879:string)  [unwired: 3 in, 3 out]
              n1266 = local write "Numeric 11"(w878) -> ()
              n1267 = String Length(string=w879) -> (length=w881:i32)
              n1268 = Greater?(x=w881, y=1) -> (0:w877:bool)
            }
            n1269 = while {
              tunnel: w859 -> [w888]
              i -> [w884]
              stop <- w883 continue-if-true
              (unwired) TRUE ("line mode (F)")
              n1270 = Read from Text File "Read File"(file (use dialog)=w888) -> (text=w885:string)  [unwired: 3 in, 3 out]
              n1271 = local write "Numeric 12"(w884) -> ()
              n1272 = String Length(string=w885) -> (length=w887:i32)
              n1273 = Greater?(x=w887, y=1) -> (0:w883:bool)
            }
            n1274 = while {
              tunnel: w858 -> [w894]
              i -> [w890]
              stop <- w889 continue-if-true
              (unwired) TRUE ("line mode (F)")
              n1275 = Read from Text File "Read File"(file (use dialog)=w894) -> (text=w891:string)  [unwired: 3 in, 3 out]
              n1276 = local write "Numeric 13"(w890) -> ()
              n1277 = String Length(string=w891) -> (length=w893:i32)
              n1278 = Greater?(x=w893, y=1) -> (0:w889:bool)
            }
          }
          frame #1 {
            w1046 = FALSE ("ACTUAL   MERGE")
            # "Sample Temp"
            # "ECR"
            # "COF"
            # "Time\nCOF\nFF\nTemp"
            n1279 = case shown="True" w919 {
              tunnel: [w1066 w1067] -> w920
              frame False {
                n1280 = local read "string1"() -> (w1066:string)
              }
              frame True {
                n1281 = local read "String Indicator 4"() -> (w1067:string)
              }
            }
            n1282 = local read "string1 2"() -> (w965:string)
            n1283 = local read "string1 4"() -> (w963:string)
            n1284 = local read "string1 3"() -> (w964:string)
            n1285 = String To Path(string=w963) -> (path=w1057:path)
            n1286 = String To Path(string=w965) -> (path=w1063:path)
            n1287 = String To Path(string=w920) -> (path=w1051:path)
            n1288 = Open/Create/Replace File "Open File"(file path (use dialog)=w1057) -> (refnum out=w1056:refnum<file>, error out=w1055:errorcluster)  [unwired: 5 in, 1 out]
            n1289 = Open/Create/Replace File "Open File"(file path (use dialog)=w1051) -> (refnum out=w1065:refnum<file>, error out=w1064:errorcluster)  [unwired: 5 in, 1 out]
            n1290 = Open/Create/Replace File "Open File"(file path (use dialog)=w1063) -> (refnum out=w1061:refnum<file>, error out=w1060:errorcluster)  [unwired: 5 in, 1 out]
            n1291 = String To Path(string=w964) -> (path=w1062:path)
            n1292 = local read "Numeric 8"() -> (w1050:i32)
            n1293 = Open/Create/Replace File "Open File"(file path (use dialog)=w1062) -> (refnum out=w1058:refnum<file>, error out=w1059:errorcluster)  [unwired: 5 in, 1 out]
            n1294 = local read "Numeric 13"() -> (w1049:i32)
            n1295 = local read "Numeric 11"() -> (w1047:i32)
            n1296 = local read "Numeric 12"() -> (w1048:i32)
            n1297 = for {
              N: w1047 -> [_]
              tunnel: w1061 -> [w1176]
              tunnel: w1060 -> [w1175]
              tunnel: [w1165] -> w1027 mode=indexing
              tunnel: [w1163] -> w1025 mode=indexing
              tunnel: [w1164] -> w1020 mode=indexing
              tunnel: w1046 -> [_]
              tunnel: [w1157] -> w1022 mode=indexing
              tunnel: [w1153] -> w998 mode=indexing
              tunnel: [w1149] -> w973 mode=indexing
              tunnel: [w1145] -> w954 mode=indexing
              tunnel: [w1140] -> w912 mode=indexing
              (unwired) TRUE ("line mode (F)")
              n1298 = Read from Text File "Read File"(file (use dialog)=w1176, error in=w1175) -> (text=w1141:string)  [unwired: 2 in, 3 out]
              n1299 = String Subset(string=w1141, offset (0)=0, length (rest)=14 ("length (rest)")) -> (substring=w1169:string)
              n1300 = Fract/Exp String To Number(string=w1169) -> (number=w1165:dbl)  [unwired: 3 in, 1 out]
              n1301 = local write "String 7"(w1141) -> ()
              n1302 = String Subset(string=w1141, offset (0)=15, length (rest)=9 ("length (rest)")) -> (substring=w1172:string)
              n1303 = Fract/Exp String To Number(string=w1172) -> (number=w1163:dbl)  [unwired: 3 in, 1 out]
              n1304 = String Subset(string=w1141, offset (0)=65, length (rest)=9 ("length (rest)")) -> (substring=w1158:string)
              n1305 = Fract/Exp String To Number(string=w1158) -> (number=w1161:dbl)  [unwired: 3 in, 1 out]
              n1306 = Add(x=w1161, y=0.0) -> (x+y=w1157:dbl)
              n1307 = String Subset(string=w1141, offset (0)=35, length (rest)=9 ("length (rest)")) -> (substring=w1166:string)
              n1308 = Fract/Exp String To Number(string=w1166) -> (number=w1164:dbl)  [unwired: 3 in, 1 out]
              n1309 = String Subset(string=w1141, offset (0)=45, length (rest)=9 ("length (rest)")) -> (substring=w1154:string)
              n1310 = Fract/Exp String To Number(string=w1154) -> (number=w1153:dbl)  [unwired: 3 in, 1 out]
              n1311 = String Subset(string=w1141, offset (0)=55, length (rest)=9 ("length (rest)")) -> (substring=w1152:string)
              n1312 = Fract/Exp String To Number(string=w1152) -> (number=w1149:dbl)  [unwired: 3 in, 1 out]
              n1313 = String Subset(string=w1141, offset (0)=25, length (rest)=9 ("length (rest)")) -> (substring=w1146:string)
              n1314 = Fract/Exp String To Number(string=w1146) -> (number=w1145:dbl)  [unwired: 3 in, 1 out]
              n1315 = String Subset(string=w1141, offset (0)=85, length (rest)=9 ("length (rest)")) -> (substring=w1144:string)
              n1316 = Fract/Exp String To Number(string=w1144) -> (number=w1140:dbl)  [unwired: 3 in, 1 out]
            }
            n1317 = for {
              N: w1048 -> [_]
              tunnel: w1059 -> [w1139]
              tunnel: w1058 -> [w1138]
              tunnel: [w1128] -> w1017 mode=indexing
              tunnel: [w1126] -> w1015 mode=indexing
              tunnel: [w1127] -> w1011 mode=indexing
              tunnel: w1046 -> [_]
              tunnel: [w1120] -> w1013 mode=indexing
              tunnel: [w1116] -> w995 mode=indexing
              tunnel: [w1112] -> w971 mode=indexing
              tunnel: [w1109] -> w952 mode=indexing
              tunnel: [w1105] -> w911 mode=indexing
              (unwired) 9 ("length (rest)")
              (unwired) 9 ("length (rest)")
              (unwired) TRUE ("line mode (F)")
              n1318 = Read from Text File "Read File"(file (use dialog)=w1138, error in=w1139) -> (text=w1106:string)  [unwired: 2 in, 3 out]
              n1319 = String Subset(string=w1106, offset (0)=0, length (rest)=14 ("length (rest)")) -> (substring=w1132:string)
              n1320 = Fract/Exp String To Number(string=w1132) -> (number=w1128:dbl)  [unwired: 3 in, 1 out]
              n1321 = local write "String 8"(w1106) -> ()
              n1322 = String Subset(string=w1106, offset (0)=15, length (rest)=9 ("length (rest)")) -> (substring=w1135:string)
              n1323 = Fract/Exp String To Number(string=w1135) -> (number=w1126:dbl)  [unwired: 3 in, 1 out]
              n1324 = String Subset(string=w1106, offset (0)=65, length (rest)=9 ("length (rest)")) -> (substring=w1125:string)
              n1325 = Fract/Exp String To Number(string=w1125) -> (number=w1122:dbl)  [unwired: 3 in, 1 out]
              n1326 = Add(x=w1122, y=0.0) -> (x+y=w1120:dbl)
              n1327 = String Subset(string=w1106, offset (0)=35, length (rest)=9 ("length (rest)")) -> (substring=w1129:string)
              n1328 = Fract/Exp String To Number(string=w1129) -> (number=w1127:dbl)  [unwired: 3 in, 1 out]
              n1329 = String Subset(string=w1106, offset (0)=45, length (rest)=9 ("length (rest)")) -> (substring=w1119:string)
              n1330 = Fract/Exp String To Number(string=w1119) -> (number=w1116:dbl)  [unwired: 3 in, 1 out]
              n1331 = String Subset(string=w1106, offset (0)=55, length (rest)=9 ("length (rest)")) -> (substring=w1114:string)
              n1332 = Fract/Exp String To Number(string=w1114) -> (number=w1112:dbl)  [unwired: 3 in, 1 out]
              n1333 = String Subset(string=w1106, offset (0)=25) -> (substring=w1110:string)  [unwired: 1 in]
              n1334 = Fract/Exp String To Number(string=w1110) -> (number=w1109:dbl)  [unwired: 3 in, 1 out]
              n1335 = String Subset(string=w1106, offset (0)=85) -> (substring=w1108:string)  [unwired: 1 in]
              n1336 = Fract/Exp String To Number(string=w1108) -> (number=w1105:dbl)  [unwired: 3 in, 1 out]
            }
            n1337 = for {
              N: w1049 -> [_]
              tunnel: w1056 -> [w1104]
              tunnel: w1055 -> [w1103]
              tunnel: [w1093] -> w1009 mode=indexing
              tunnel: [w1092] -> w1002 mode=indexing
              tunnel: w1046 -> [_]
              tunnel: [w1081] -> w1007 mode=indexing
              tunnel: [w1086] -> w1004 mode=indexing
              tunnel: [w1082] -> w994 mode=indexing
              tunnel: [w1077] -> w969 mode=indexing
              tunnel: [w1073] -> w950 mode=indexing
              tunnel: [w1068] -> w910 mode=indexing
              (unwired) 1.0 ("x")
              (unwired) TRUE ("line mode (F)")
              n1338 = Read from Text File "Read File"(file (use dialog)=w1104, error in=w1103) -> (text=w1069:string)  [unwired: 2 in, 3 out]
              n1339 = String Subset(string=w1069, offset (0)=0, length (rest)=14 ("length (rest)")) -> (substring=w1097:string)
              n1340 = Fract/Exp String To Number(string=w1097) -> (number=w1093:dbl)  [unwired: 3 in, 1 out]
              n1341 = String Subset(string=w1069, offset (0)=15, length (rest)=9 ("length (rest)")) -> (substring=w1100:string)
              n1342 = local write "String 12"(w1069) -> ()
              n1343 = Fract/Exp String To Number(string=w1100) -> (number=w1081:dbl)  [unwired: 3 in, 1 out]
              n1344 = String Subset(string=w1069, offset (0)=65, length (rest)=9 ("length (rest)")) -> (substring=w1087:string)
              n1345 = Fract/Exp String To Number(string=w1087) -> (number=w1090:dbl)  [unwired: 3 in, 1 out]
              n1346 = Add(x=w1090, y=0.0) -> (x+y=w1086:dbl)
              n1347 = String Subset(string=w1069, offset (0)=35, length (rest)=9 ("length (rest)")) -> (substring=w1094:string)
              n1348 = Fract/Exp String To Number(string=w1094) -> (number=w1092:dbl)  [unwired: 3 in, 1 out]
              n1349 = String Subset(string=w1069, offset (0)=45, length (rest)=9 ("length (rest)")) -> (substring=w1084:string)
              n1350 = Fract/Exp String To Number(string=w1084) -> (number=w1082:dbl)  [unwired: 3 in, 1 out]
              n1351 = String Subset(string=w1069, offset (0)=55, length (rest)=9 ("length (rest)")) -> (substring=w1079:string)
              n1352 = Fract/Exp String To Number(string=w1079) -> (number=w1077:dbl)  [unwired: 3 in, 1 out]
              n1353 = String Subset(string=w1069, offset (0)=25, length (rest)=9 ("length (rest)")) -> (substring=w1075:string)
              n1354 = Fract/Exp String To Number(string=w1075) -> (number=w1073:dbl)  [unwired: 3 in, 1 out]
              n1355 = String Subset(string=w1069, offset (0)=85, length (rest)=9 ("length (rest)")) -> (substring=w1071:string)
              n1356 = Fract/Exp String To Number(string=w1071) -> (number=w1068:dbl)  [unwired: 3 in, 1 out]
            }
            n1357 = for {
              N: w1050 -> [_]
              tunnel: w1065 -> [w1213]
              tunnel: w1064 -> [w1212]
              tunnel: [w1202] -> w977 mode=indexing
              tunnel: [w1200] -> w1034 mode=indexing
              tunnel: [w1201] -> w1029 mode=indexing
              tunnel: w1046 -> [_]
              tunnel: [w1194] -> w1031 mode=indexing
              tunnel: [w1190] -> w1000 mode=indexing
              tunnel: [w1186] -> w975 mode=indexing
              tunnel: [w1182] -> w956 mode=indexing
              tunnel: [w1177] -> w916 mode=indexing
              (unwired) TRUE ("line mode (F)")
              # "freq"
              # "Stroke"
              # "Time"
              # "CoF"
              # "Humidity"
              # "Temp"
              # "Air Temp"
              # "ECR"
              n1358 = Read from Text File "Read File"(file (use dialog)=w1213, error in=w1212) -> (text=w1178:string)  [unwired: 2 in, 3 out]
              n1359 = String Subset(string=w1178, offset (0)=0, length (rest)=14 ("length (rest)")) -> (substring=w1206:string)
              n1360 = Fract/Exp String To Number(string=w1206) -> (number=w1202:dbl)  [unwired: 3 in, 1 out]
              n1361 = local write "String 6"(w1178) -> ()
              n1362 = String Subset(string=w1178, offset (0)=15, length (rest)=9 ("length (rest)")) -> (substring=w1209:string)
              n1363 = Fract/Exp String To Number(string=w1209) -> (number=w1200:dbl)  [unwired: 3 in, 1 out]
              n1364 = String Subset(string=w1178, offset (0)=65, length (rest)=9 ("length (rest)")) -> (substring=w1199:string)
              n1365 = Fract/Exp String To Number(string=w1199) -> (number=w1196:dbl)  [unwired: 3 in, 1 out]
              n1366 = Add(x=w1196, y=0.0) -> (x+y=w1194:dbl)
              n1367 = String Subset(string=w1178, offset (0)=35, length (rest)=9 ("length (rest)")) -> (substring=w1203:string)
              n1368 = Fract/Exp String To Number(string=w1203) -> (number=w1201:dbl)  [unwired: 3 in, 1 out]
